vi "udp.ip.reader.vi"(6 "IP Address":T2=[176, 197, 84, 255], 7 "MAC Address":T1=[176, 197, 84, 255, 244, 135] format="%.0x", 8 "Dest Port":u16, 9 "end_of_frame":bool, 10 "data_valid":bool, 11 "data":u8) -> (1 "udp_byte_enable":bool, 2 "udp_data valid_out":bool, 3 "udp_data_out":u8)   [LabVIEW 2022 SP3]
uses:
  <instrlib>/_niInstr/Network/Types/v1/IPv4 Address.ctl
  <instrlib>/_niInstr/Network/Types/v1/MAC Address.ctl
  <instrlib>/_niInstr/Network/IPv4/UDP/Data Stream/v1/Read Data Stream.vi
  <instrlib>/_niInstr/Network/IPv4/FPGA/v1/niInstr IPv4 FPGA v1.lvlib
  <instrlib>/_niInstr/Network/IPv4/UDP/FPGA/v1/niInstr IPv4 UDP FPGA v1.lvlib
  <instrlib>/_niInstr/Network/Ethernet/Utility/v1/FPGA/niInstr Ethernet Utilities FPGA v1.lvlib
  <instrlib>/_niInstr/Network/IPv4/UDP/Data Stream/v1/niInstr IPv4 UDP Data Stream v1.lvclass
  <instrlib>/_niInstr/Network/Types/v1/niInstr Network Types v1.lvlib
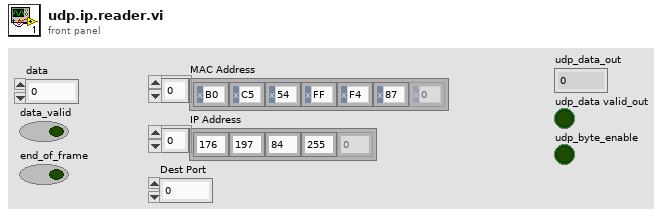
[diagram p1: front panel]
types:
  T1 = typedef "niInstr Network Types v1.lvlib/MAC Address.ctl" = u8[]
  T2 = typedef "niInstr Network Types v1.lvlib/IPv4 Address.ctl" = u8[]
  T3 = typedef "niInstr Ethernet Utilities FPGA v1.lvlib/Network Data Stream.ctl" = cluster{"data":u8[], "data valid":bool, "byte enables":bool[]}
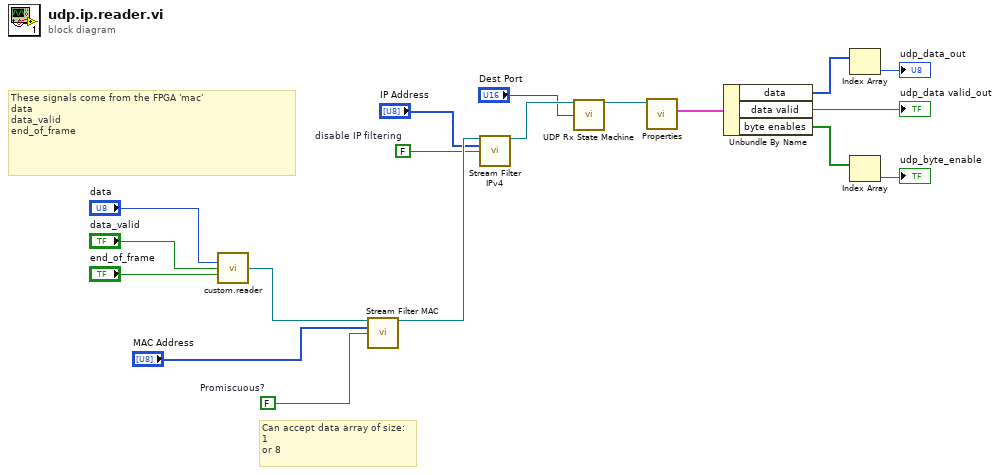
[diagram p0: block diagram]
diagram:
  w16 = FALSE  # disable IP filtering
  w15 = FALSE  # Promiscuous?
  # "These signals come from the FPGA 'mac'\ndata\ndata_valid\nend_of_frame"
  # "Can accept data array of size:\n1\nor 8"
  n1 = call "custom.reader.vi"("data"="data", "data_valid"="data_valid", "end_of_frame"="end_of_frame") -> ("niInstr Ethernet MAC Raw Stream v1.lvclass"=w12:refnum<class "niInstr Ethernet MAC Raw Stream v1.lvclass">)  [unwired: 12 in]
  n2 = call <instrlib>:"Stream Filter MAC.vi"("niInstr Ethernet MAC Raw Stream v1 in"=w12, "MAC Address"="MAC Address", "Promiscuous?"=w15) -> ("niInstr Ethernet MAC Data Stream v1 out"=w17:refnum<class "niInstr Ethernet MAC Data Stream v1.lvclass">)  [unwired: 12 in]
  n3 = call <instrlib>:"Stream Filter IPv4.vi"("niInstr Ethernet MAC Data Stream v1 in"=w17, "IP Address"="IP Address", "disable IP filtering"=w16) -> ("niInstr IPv4 Data Stream out"=w18:refnum<class "niInstr IPv4 Data Stream v1.lvclass">)  [unwired: 12 in]
  n4 = call <instrlib>:"UDP Rx State Machine.vi"("niInstr IPv4 Data Stream in"=w18, "Dest Port"="Dest Port") -> ("niInstr IPv4 UDP Data Stream out"=w14:refnum<class "niInstr IPv4 UDP Data Stream v1.lvclass">)  [unwired: 13 in]
  n5 = call-poly <instrlib>:"Properties.vi"("niInstr IPv4 UDP Data Stream v1.lvclass"=w14) -> ("Data Stream"=w13:T3)  [unwired: 9 in, 1 out]
  n6 = Unbundle By Name(w13) -> ("data"=w7:u8[], "data valid"=→"udp_data valid_out":bool, "byte enables"=w5:bool[])
  n7 = Index Array(array=w7) -> (element=→"udp_data_out":u8)  [unwired: 1 in]
  n8 = Index Array(array=w5) -> (element=→"udp_byte_enable":bool)  [unwired: 1 in]
